vi "moveToGetPointsFromRAM2.vi"(5 "Memory In":refnum<k21>="moveToWave", 6 "inputValid":bool=TRUE, 7 "reset":bool=TRUE, 8 "maxReached":bool, 9 "interpPosition":fxp<+,16,0>, 11 "adresses":cluster{"currentPoint":u16, "nextPoint":u16}) -> (0 "outputValid":bool=TRUE, 3 "interpOutput":fxp<+/-,19,2>)   [LabVIEW 2016]
uses:
  <vilib>/rvi/Emulation/niFpgaSctlEmulationGetInTimedLoop.vi
  <vilib>/Utility/error.llb/Clear Errors.vi
  <vilib>/rvi/DataTransferAndStorage/Container/Common/niFpgaContainerExecOnDevCompGetState.vi
  <vilib>/rvi/Emulation/niFpgaEmulationIsFPGAContextNoSignature.vi
  <vilib>/rvi/DataTransferAndStorage/Container/Common/niFpgaContainerGetUniqueNameForEmu.vi
  <vilib>/rvi/Emulation/niFpgaProcessEmulError.vi
  <vilib>/rvi/errors/nirviReportUnexpectedCaseInternalError (U32).vi
  <vilib>/rvi/Memory/Memory_Emulation/niFpgaMemoryEmulationCacheClearOnFirstRun.vi
  <vilib>/rvi/Memory/Memory_Emulation/nirvimemoryEmulationManagerCache_MakeExclusive.vi
  <vilib>/rvi/Memory/Memory_Emulation/niFpgaMemoryEmulationValidateCache.vi
  <vilib>/rvi/Memory/Memory_Emulation/nirvimemoryEmulationManagerCache_InsertValue.vi
  <vilib>/rvi/Memory/Memory_Emulation/nirvimemoryEmulationManagerCache_ReleaseExclusive.vi
  <vilib>/rvi/Memory/Memory_Emulation/nirvimemoryEmulationManagerCache_GetValue.vi
  <vilib>/rvi/Memory/Memory_Emulation/nirvimemoryEmulationManagerCache_SetValue.vi
  <vilib>/rvi/Emulation/niFpgaSctlEmulationResourceMgr.vi
  <vilib>/rvi/Analysis/common/FxpNativeNode/niFpgaFxpNative.xnode
  <vilib>/rvi/DataTransferAndStorage/Container/XNode/niFpgaContainer.xnode
  <vilib>/rvi/Memory/Memory_Emulation/niFpgaMemoryEmulationRefIn.vi
  <instrlib>/_niInstr/Basic Elements/v1/FPGA/niInstr Basic Elements v1 FPGA.lvlib
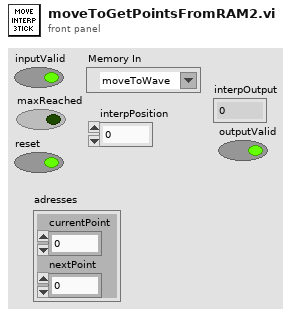
[diagram p1: front panel]
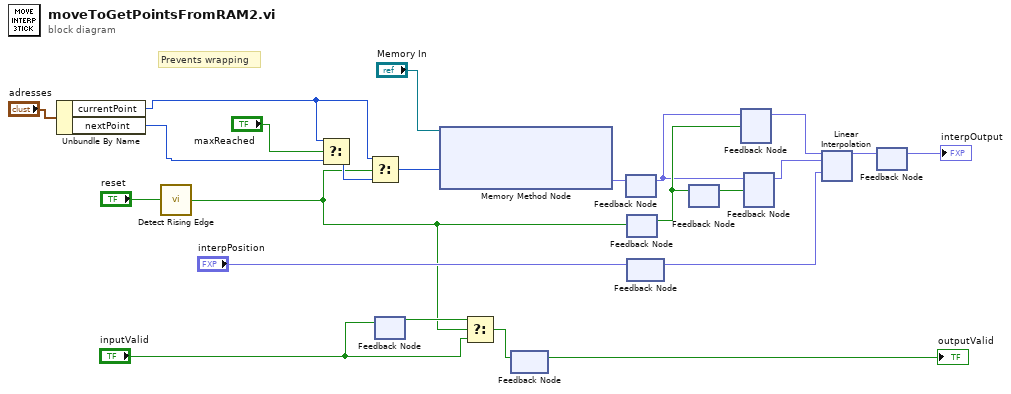
[diagram p0: block diagram]
diagram:
  # "Prevents wrapping"
  n1 = Unbundle By Name("adresses") -> ("currentPoint"=w7:u16, "nextPoint"=w6:u16)
  n2 = call <instrlib>:"Detect Rising Edge.vi"("signal"="reset") -> ("edge detected"=w2:bool)  [unwired: 14 in]
  n3 = Select(t=w7, s="maxReached", f=w6) -> (s? t:f=w20:u16)
  n4 = Select(t=w7, s=w2, f=w20) -> (s? t:f=w21:u16)
  n5 = feedback #1() -> (w4:bool)  [unwired: 1 in]
  n6 = feedback-in #1("inputValid") -> ()
  n7 = xnode ("Memory Method Node")("Address"=w21, "Memory In"="Memory In") -> ("Data"=w22:fxp<+/-,19,2>)  [unwired: 1 out]
  n8 = Select(t=w4, s=w2, f="inputValid") -> (s? t:f=w1:bool)
  n9 = feedback-in #2(w1) -> ()
  n10 = feedback #2() -> (→"outputValid":bool)  [unwired: 1 in]
  n11 = feedback #3() -> (w16:fxp<+/-,19,2>)  [unwired: 1 in]
  n12 = feedback-in #3(w22) -> ()
  n13 = feedback #4() -> (w19:bool)  [unwired: 1 in]
  n14 = feedback-in #4(w2) -> ()
  n15 = feedback #5() -> (w23:fxp<+,16,0>)  [unwired: 1 in]
  n16 = feedback-in #5("interpPosition") -> ()
  n17 = feedback #6() -> (w17:bool)  [unwired: 1 in]
  n18 = feedback-in #6(w19) -> ()
  n19 = feedback #7() -> (w18:fxp<+/-,19,2>)  [unwired: 1 in]
  n20 = feedback-in #7(w16, w19) -> ()
  n21 = feedback #8() -> (w15:fxp<+/-,19,2>)  [unwired: 1 in]
  n22 = feedback-in #8(w16, w17) -> ()
  n23 = xnode ("Linear Interpolation")("y0"=w18, "y1"=w15, "x"=w23) -> ("y"=w12:fxp<+/-,19,2>)
  n24 = feedback-in #9(w12) -> ()
  n25 = feedback #9() -> (→"interpOutput":fxp<+/-,19,2>)  [unwired: 1 in]
